vi "TEST Object Manual Bounds (Interactive Splitter).vi"() -> ()   [LabVIEW 2021, in "IObject.lvclass"]
uses:
  IObject.lvclass
  Object/Object.lvclass
  C:/Projects/Dynamic-Scaling/Dynamic Scaling/IObject.lvclass
  IContainer/Viewport/Viewport.lvclass
  IContainer/Divider/Splitter/Splitter.lvclass
  IContainer/Interaction/Interaction.lvclass
panel:
  out "XY Graph 3":cluster{"X":dbl, "Y":dbl}[](graph)
  out "XY Graph 2":cluster{"X":dbl, "Y":dbl}[](graph)
  out "XY Graph":cluster{"X":dbl, "Y":dbl}[](graph)
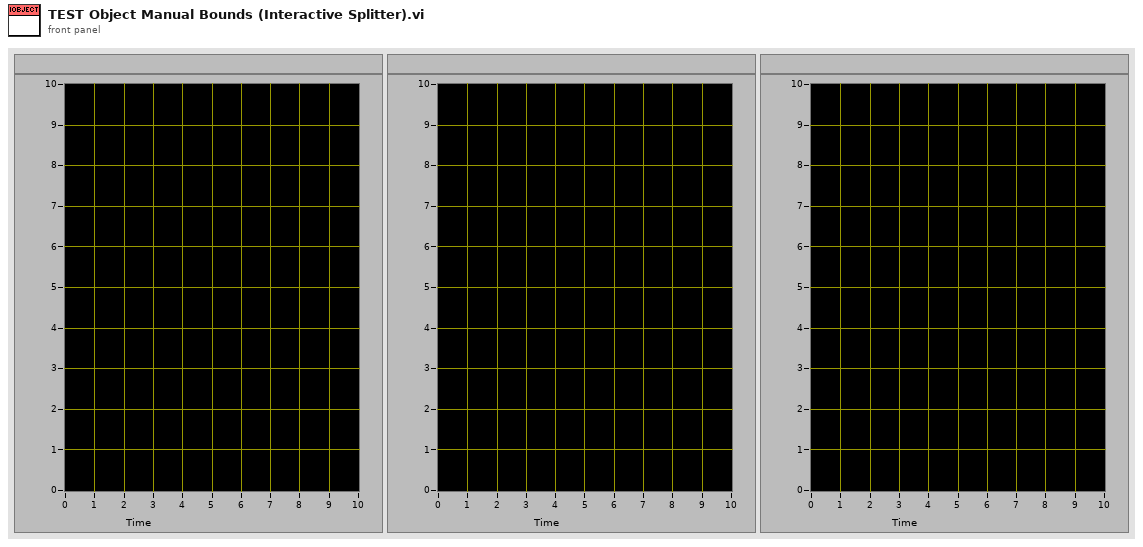
[diagram p1: front panel]
types:
  T1 = cluster{"Left":dbl, "Top":dbl, "Right":dbl, "Bottom":dbl}
  T2 = typedef "LVRectTypeDef.ctl" = cluster{"Left":i16, "Top":i16, "Right":i16, "Bottom":i16}
  T3 = typedef "LVPoint32TypeDef.ctl" = cluster{"Horizontal":i32, "Vertical":i32}
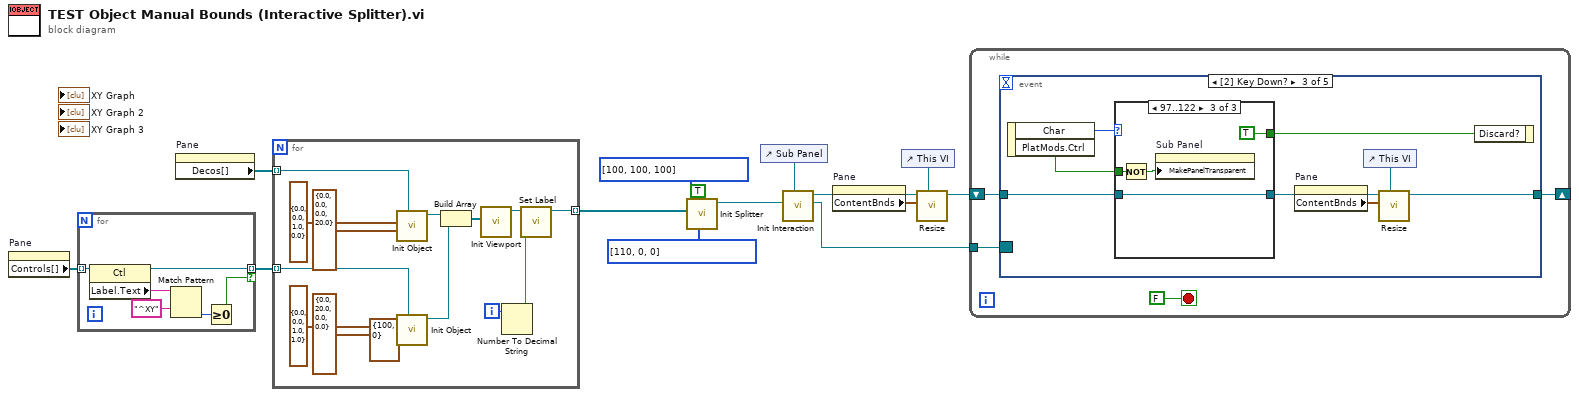
[diagram p0: block diagram]
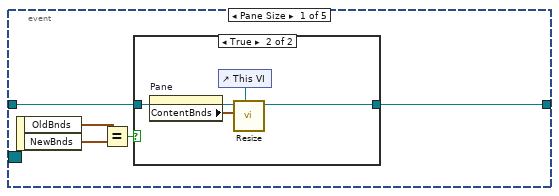
[diagram p2: hidden frame]
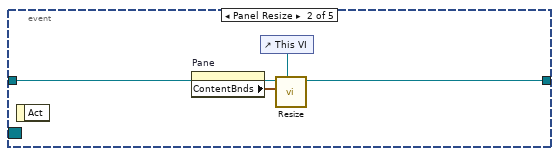
[diagram p4: hidden frame]
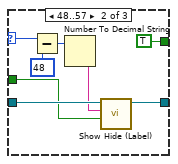
[diagram p6: hidden frame]
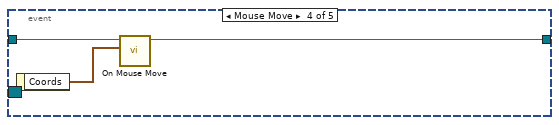
[diagram p7: hidden frame]
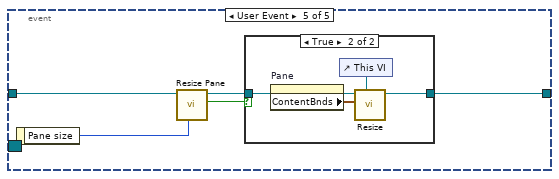
[diagram p8: hidden frame]
diagram:
  n1 = property on="Pane" class="Pane"() -> ("Controls[]"=w10:refnum<vi>[])  [unwired: 2 in, 2 out]
  n2 = for {
    tunnel: w10 -> [w20] mode=indexing
    tunnel: [w17] -> w9 mode=indexing if=w15
    n3 = property class="Ctl"(reference=w20) -> (reference out=w17:refnum<vi>, "Label.Text"=w19:string)  [unwired: 1 in, 1 out]
    n4 = Match Pattern(string=w19, regular expression="^XY") -> (offset past match=w16:i32)  [unwired: 1 in, 3 out]
    n5 = Greater Or Equal To 0?(x=w16) -> (x >= 0?=w15:bool)
  }
  n6 = property on="Pane" class="Pane"() -> ("Decos[]"=w14:refnum<vi>[])  [unwired: 2 in, 2 out]
  n7 = for {
    tunnel: w14 -> [w34] mode=indexing
    tunnel: [w23] -> w2 mode=indexing
    tunnel: w9 -> [w27] mode=indexing
    i -> [w33]
    n8 = call "Init Object.vi"("GObj Refnum"=w34, "B [0, 0, 0, 0]"=T1 {"Left"=0.0, "Top"=0.0, "Right"=0.0, "Bottom"=20.0} ("B"), "A [0, 0, 1, 1]"=T1 {"Left"=0.0, "Top"=0.0, "Right"=1.0, "Bottom"=0.0} ("A")) -> ("MMI Scaling out"=w25:refnum<class "Object.lvclass">)  [unwired: 7 in, 1 out]
    n9 = call "Init Object.vi"("Minimal size [0, 0]"=cluster{"Horizontal":i16, "Vertical":i16} {"Horizontal"=100, "Vertical"=0}, "GObj Refnum"=w27, "B [0, 0, 0, 0]"=T1 {"Left"=0.0, "Top"=20.0, "Right"=0.0, "Bottom"=0.0} ("B"), "A [0, 0, 1, 1]"=T1 {"Left"=0.0, "Top"=0.0, "Right"=1.0, "Bottom"=1.0} ("A")) -> ("MMI Scaling out"=w24:refnum<class "Object.lvclass">)  [unwired: 6 in, 1 out]
    n10 = Build Array(w25, w24) -> (w30:refnum<class "Object.lvclass">[])
    n11 = call "Init Viewport.vi"("Items"=w30) -> ("Viewport out"=w22:refnum<class "Viewport.lvclass">)  [unwired: 9 in, 1 out]
    n12 = Number To Decimal String(number=w33) -> (decimal integer string=w26:string)  [unwired: 1 in]
    n13 = call "Set Label.vi"("Label"=w26, "MMI Scaling in"=w22) -> ("MMI Scaling out"=w23:refnum<class "Viewport.lvclass">)  [unwired: 8 in, 1 out]
  }
  n14 = call "Init Splitter.vi"("Minimal size"=i16[] [110, 0, 0], "Vertical? [F, hor.]"=TRUE, "Relative size"=i16[] [100, 100, 100] ("Minimal size"), "Items"=w2) -> ("Splitter out"=w1:refnum<class "Splitter.lvclass">)  [unwired: 6 in, 1 out]
  n15 = control-ref of="Sub Panel"() -> (w8:refnum<vi>)
  n16 = call "Init Interaction.vi"("Sub Panel"=w8, "IObject"=w1) -> ("Interaction Splitter Resize"=w3:refnum<event-registration>, "Interaction out"=w5:refnum<class "Interaction.lvclass">)  [unwired: 6 in, 2 out]
  n17 = property on="Pane" class="Pane"() -> ("ContentBnds"=w6:T2)  [unwired: 2 in, 2 out]
  n18 = control-ref of="This VI"() -> (w7:refnum<vi>)
  n19 = call-dynamic "Resize.vi"("VI Refnum"=w7, "Bounds"=w6, "MMI Scaling in"=w5) -> ("MMI Scaling out"=w4:refnum<class "Interaction.lvclass">)  [unwired: 6 in, 2 out]
  n20 = while {
    shift-right: [w36] -> _
    shift-left: w4 -> [w38]
    tunnel: w3 -> [w35]
    stop <- FALSE stop-if-true
    n21 = event shown="[2] Key Down?" {
      selector: w35 -> [_ _ _ _ _]
      dyn-events: _ -> [_ _ _ _ _]
      timeout: _ -> [_ _ _ _ _]
      tunnel: w38 -> [w43 w52 w56 w76 w81]
      tunnel: [w42 w51 w54 w75 w77] -> w36
      event Pane Size {
        n22 = event-data() -> ("OldBnds"=w41:T2, "NewBnds"=w40:T2)  [unwired: 1 in]
        n23 = Equal?(x=w41, y=w40) -> (x = y?=w39:bool)
        n24 = case shown="True" w39 {
          tunnel: w43 -> [w44 w48]
          tunnel: [w44 w45] -> w42
          frame False {
          }
          frame True {
            n25 = property on="Pane" class="Pane"() -> ("ContentBnds"=w47:T2)  [unwired: 2 in, 2 out]
            n26 = control-ref of="This VI"() -> (w46:refnum<vi>)
            n27 = call-dynamic "Resize.vi"("VI Refnum"=w46, "Bounds"=w47, "MMI Scaling in"=w48) -> ("MMI Scaling out"=w45:refnum<class "Interaction.lvclass">)  [unwired: 6 in, 2 out]
          }
        }
      }
      event Panel Resize {
        n28 = event-data() -> ()  [unwired: 1 in, 1 out]
        n29 = property on="Pane" class="Pane"() -> ("ContentBnds"=w50:T2)  [unwired: 2 in, 2 out]
        n30 = control-ref of="This VI"() -> (w49:refnum<vi>)
        n31 = call-dynamic "Resize.vi"("VI Refnum"=w49, "Bounds"=w50, "MMI Scaling in"=w52) -> ("MMI Scaling out"=w51:refnum<class "Interaction.lvclass">)  [unwired: 6 in, 2 out]
      }
      event Key Down? {
        n32 = event-data() -> ("Char"=w58:i16, "PlatMods.Ctrl"=w55:bool)  [unwired: 1 in]
        n33 = case shown="97..122" w58 {
          selector: w58 -> [_ w69 _]
          tunnel: [w61 w65 w72] -> w57
          tunnel: w56 -> [w61 w67 w72]
          tunnel: w55 -> [_ w64 w71]
          tunnel: [_ TRUE TRUE] -> w53
          frame Default {
          }
          frame 48..57 {
            n34 = Subtract(x=w69, y=i16 48) -> (x-y=w66:i16)
            n35 = Number To Decimal String(number=w66) -> (decimal integer string=w63:string)  [unwired: 1 in]
            n36 = call-dynamic "Show Hide (Label).vi"("Show? [T]"=w64, "Label"=w63, "MMI Scaling in"=w67) -> ("MMI Scaling out"=w65:refnum<class "Interaction.lvclass">)  [unwired: 6 in, 2 out]
          }
          frame 97..122 {
            n37 = Not(x=w71) -> (.not. x?=w70:bool)
            n38 = property on="Sub Panel" class="SubPnl"("MakePanelTransparent"=w70) -> ()  [unwired: 2 in, 2 out]
          }
        }
        n39 = property on="Pane" class="Pane"() -> ("ContentBnds"=w60:T2)  [unwired: 2 in, 2 out]
        n40 = control-ref of="This VI"() -> (w59:refnum<vi>)
        n41 = call-dynamic "Resize.vi"("VI Refnum"=w59, "Bounds"=w60, "MMI Scaling in"=w57) -> ("MMI Scaling out"=w54:refnum<class "Interaction.lvclass">)  [unwired: 6 in, 2 out]
        n42 = event-data("Discard?"=w53) -> ()  [unwired: 1 in, 1 out]
      }
      event Mouse Move {
        n43 = event-data() -> ("Coords"=w74:T3)  [unwired: 1 in]
        n44 = call "On Mouse Move.vi"("Coords"=w74, "Interaction in"=w76) -> ("Interaction out"=w75:refnum<class "Interaction.lvclass">)  [unwired: 8 in, 1 out]
      }
      event User Event {
        n45 = event-data() -> ("Pane size"=w80:i32)  [unwired: 1 in]
        n46 = call-dynamic "Resize Pane.vi"("Pane size"=w80, "IContainer in"=w81) -> ("Resized?"=w79:bool, "IContainer out"=w78:refnum<class "Interaction.lvclass">)  [unwired: 7 in, 1 out]
        n47 = case shown="True" w79 {
          tunnel: [w82 w84] -> w77
          tunnel: w78 -> [w82 w83]
          frame False {
          }
          frame True {
            n48 = property on="Pane" class="Pane"() -> ("ContentBnds"=w86:T2)  [unwired: 2 in, 2 out]
            n49 = control-ref of="This VI"() -> (w85:refnum<vi>)
            n50 = call-dynamic "Resize.vi"("VI Refnum"=w85, "Bounds"=w86, "MMI Scaling in"=w83) -> ("MMI Scaling out"=w84:refnum<class "Interaction.lvclass">)  [unwired: 6 in, 2 out]
          }
        }
      }
    }
  }
